vi "rlc.vi"(0 "LstBox Refnum":refnum<vi>, 1 "F values array":dbl[][](array[numeric]), 6 "Frekanslar":dbl[](array[numeric]), 7 "frekans index":dbl) -> (14 "10R values":dbl, 15 "1R values":dbl)   [LabVIEW 2014]
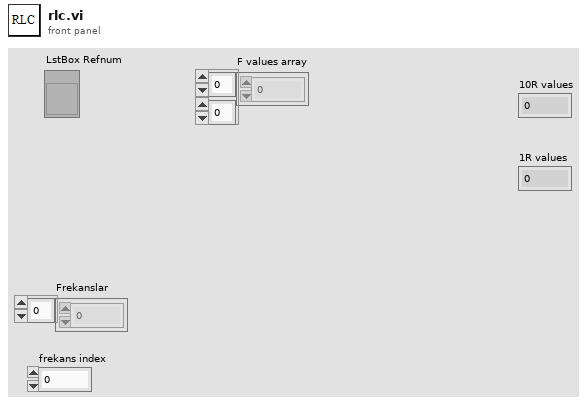
[diagram p1: front panel]
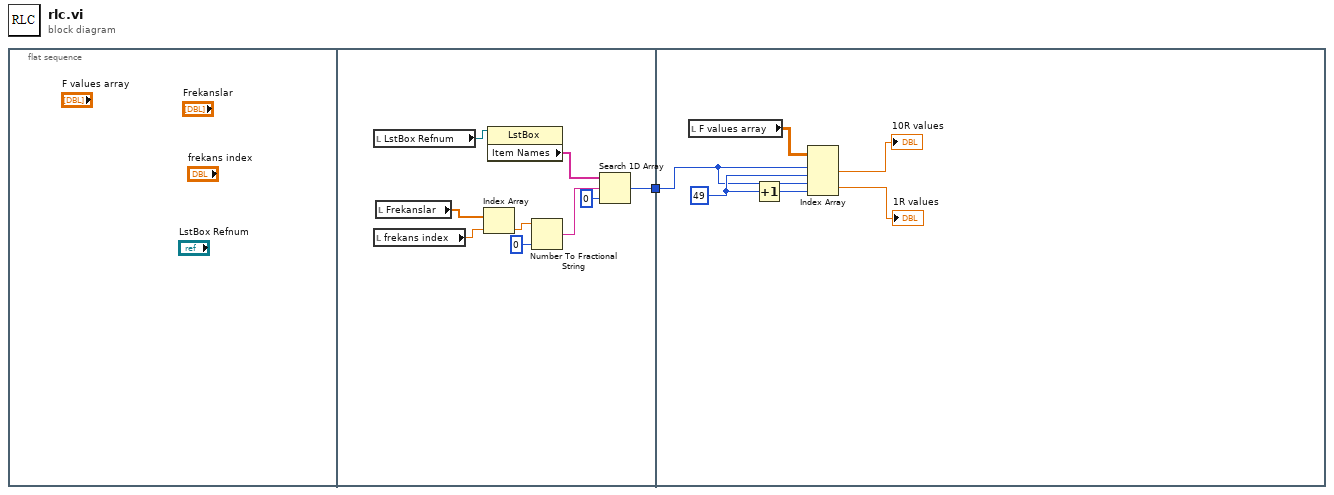
[diagram p0: block diagram]
diagram:
  n1 = flat-sequence {
    tunnel: [w2] -> w1
    tunnel: w1 -> [w14]
    frame #0 {
    }
    frame #1 {
      n2 = local read "LstBox Refnum"() -> (w10:refnum<vi>)
      n3 = local read "frekans index"() -> (w8:dbl)
      n4 = local read "Frekanslar"() -> (w9:dbl[])
      n5 = Index Array(array=w9, index=w8) -> (element=w7:dbl)
      n6 = property class="LstBox"(reference=w10) -> ("Item Names"=w6:string[])  [unwired: 1 in, 2 out]
      n7 = Number To Fractional String(number=w7, precision (6)=i16 0) -> (F-format string=w5:string)  [unwired: 2 in]
      n8 = Search 1D Array(1D array=w6, element=w5, start index (0)=0) -> (index of element=w2:i32)
    }
    frame #2 {
      w15 = 49 ("disabled index (col)")
      n9 = local read "F values array"() -> (w16:dbl[][])
      n10 = Increment(x=w15) -> (x+1=w13:i32)
      n11 = Index Array(array=w16, index (row) #1=w14, index (col) #1=w15, index (row) #2=w14, index (col) #2=w13) -> (element #1=→"10R values":dbl, element #2=→"1R values":dbl)
    }
  }
